vi "Main Data Log.vi"(8 "error in (no error)":errorcluster, 11 "main ref":T1) -> (0 "error out":errorcluster)   [LabVIEW 2025]
uses:
  controls/LAB-IQ UI Data.ctl
  Traction Loop/Traction Receipe Enum.ctl
panel:
  out "error out 2":errorcluster
  out "TDMS CLOSE":bool
  out "tdms file out":refnum<k34>
  out "File Create Temp":bool
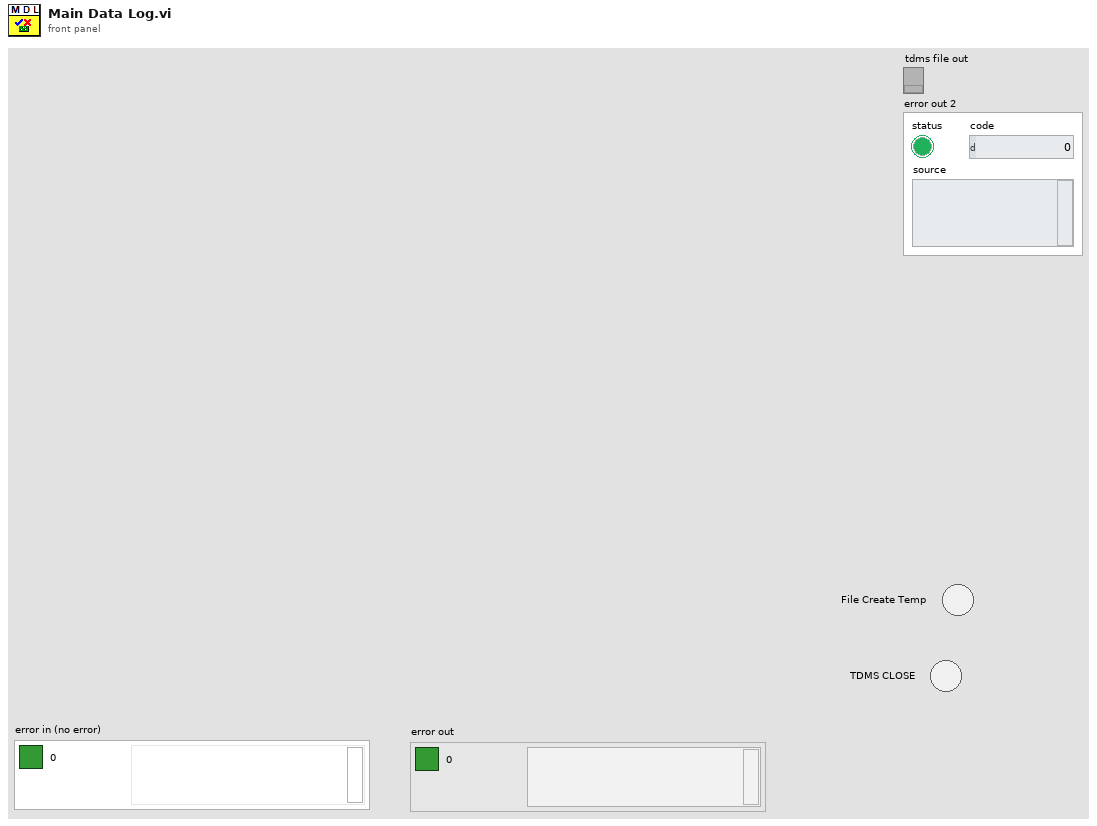
[diagram p1: front panel]
types:
  T1 = typedef "LAB-IQ UI Data.ctl" = cluster{"Main Home Screen":cluster{"GUI":refnum<vi>, "Platform Settings":refnum<vi>, "Configure":refnum<vi>, "Home":refnum<vi>, "EXIT":refnum<vi>, "service 2":refnum<vi>, "MainPage":refnum<vi>, "Analysis":refnum<vi>}, "Platform Settings":cluster{"mm/s  Surge":refnum<vi>, "Drive Error":refnum<vi>, "Disable Axis Jog Soft Limits":refnum<vi>, "mm/s  Sway":refnum<vi>, "Sway and Surge COM Status":refnum<vi>, "Heave COM Status":refnum<vi>, "Enable Platform":refnum<vi>, "Surge Forward Main":refnum<vi>, "Sway Right Main":refnum<vi>, "Sway Left Main":refnum<vi>, "Heave Down Main":refnum<vi>, "Heave Up main":refnum<vi>, "mm/s Heave":refnum<vi>, "mm/sec":refnum<vi>, "mm":refnum<vi>, "Surge Backward Main":refnum<vi>}, "Analysis Screen":cluster{"Analysis Home":refnum<vi>, "Surface Analysis":refnum<vi>, "Imaging":refnum<vi>, "Image Analysis":refnum<vi>, "Post Analysis":refnum<vi>}, "Config Screen":cluster{"Select Load Head":refnum<vi>, "Notes :":refnum<vi>, "FILE":refnum<vi>, "Sample ID :":refnum<vi>, "Operator ID :":refnum<vi>, "Operator Name :":refnum<vi>, "Auto":refnum<vi>}, "Motion Module":cluster{"zNL":refnum<vi>, "NL disp":refnum<vi>, "Rotary Tab":refnum<vi>, "Motion Direction:  3":refnum<vi>, "E.Velocity 2":refnum<vi>, "e.v/ssr 2":refnum<vi>, "Enter Fixed E.Velocity 2":refnum<vi>, "Enter Final SRR 2":refnum<vi>, "Enter initial SRR 2":refnum<vi>, "Enter Fixed SRR 2":refnum<vi>, "Enter the Final E.Velocity (m/s) 2":refnum<vi>, "Enter initial E.Velocity (m/s) 2":refnum<vi>, "Final Speed (RPM) 3":refnum<vi>, "Initial Speed (RPM) 2":refnum<vi>, "Enter the Final Velocity (m/s) 3":refnum<vi>, "Enter initial Velocity (m/s)  3":refnum<vi>, "Ramp Up 2":refnum<vi>, "TEST SELECTION":refnum<vi>, "SPEED SELECTION : ":refnum<vi>, "Angular Oscillation Set":refnum<vi>, "Traction":refnum<vi>, "Step Speed":refnum<vi>, "StepTable For Load-Speed":refnum<vi>, "StepTable For Speed":refnum<vi>, "Surge Forward MM":refnum<vi>, "Surge Backward MM":refnum<vi>, "M3 Image":refnum<vi>, "String 39":refnum<vi>, "Sway Left MM":refnum<vi>, "Sway Right MM":refnum<vi>, "Disable Axis Jog Soft Limits":refnum<vi>, "mm":refnum<vi>, "Heave Down MM":refnum<vi>, "Heave Up MM":refnum<vi>, "Wear Track Diameter (mm)":refnum<vi>, "Set WTD":refnum<vi>, "HomeScratch":refnum<vi>, "HomeRot":refnum<vi>, "PlaceModule":refnum<vi>, "Enter the Angle (Deg)":refnum<vi>, "Enter the Frequency (Hz)":refnum<vi>, "Motion Mode:":refnum<vi>, "LR Sway":refnum<vi>, "Rot Hor":refnum<vi>, "Scratch":refnum<vi>, "LR Cam":refnum<vi>, "MMBack":refnum<vi>, "MMNext":refnum<vi>, "Rot Ver":refnum<vi>, "Rotary Module Selection":refnum<vi>, "calculate rotary":refnum<vi>, "SPEED SELECTION : rotary":refnum<vi>, "Import 2":refnum<vi>, "Save 2":refnum<vi>, "File Path :  2":refnum<vi>, "String 45":refnum<vi>, "StepTable For Speed 3":refnum<vi>, "Enter the Speed(mm/sec)":refnum<vi>, "Enter the Speed(RPM)":refnum<vi>, "Enter Scratch Speed (mm/s):":refnum<vi>, "SwaySpeed Set":refnum<vi>, "Scartch Offset":refnum<vi>, "Motion type:":refnum<vi>, "HomeScratch 2":refnum<vi>, "Enter Scratch length (mm):":refnum<vi>, "Wear Track Diameter":refnum<vi>, "Rotary Speed Exced":refnum<vi>, "Scratch Mode":refnum<vi>, "No of Scratch":refnum<vi>}, "Environmental control":cluster{"Humidity  Status  3":refnum<vi>, "Low Temp  Status  2":refnum<vi>, "TK4 status 2":refnum<vi>, "Stage Temperature":refnum<vi>, "Sample Temperature":refnum<vi>, "Humidity (Amb)":refnum<vi>, "Clear List":refnum<vi>, "Add to list":refnum<vi>, "Wear":refnum<vi>, "Vibration":refnum<vi>, "Humidity (Chamber)":refnum<vi>, "Temperature (Chamber)":refnum<vi>, "ECR ":refnum<vi>, "Temperature (Amb)":refnum<vi>, "Microphone":refnum<vi>, "Acoustic Emission 3":refnum<vi>, "SNext":refnum<vi>, "APBack":refnum<vi>, "Enter the Temperature (°C):":refnum<vi>, "Enter the Stage \nTemperature (°C):":refnum<vi>, "Enter the Humidity (%Rh):":refnum<vi>, "Low Temp":refnum<vi>, "High Temp":refnum<vi>, "Humidity":refnum<vi>, "Sensors Picked":refnum<vi>}, "About Screen":cluster{"Password":refnum<vi>, "Home Service":refnum<vi>, "Advanced Setting":refnum<vi>, "About Tab":refnum<vi>, "ECR Port:":refnum<vi>, "Ramp Port:":refnum<vi>, "Installation/Replacement completed":refnum<vi>, "Loahead":refnum<vi>, "Heave and Surge COM Port:":refnum<vi>, "Sway COM Port:":refnum<vi>, "Temp Modbus:":refnum<vi>, "Humidity Port:":refnum<vi>, "Edit Gain Constants":refnum<vi>, "Save Gain Constants":refnum<vi>}, "Main Screen":cluster{"Main Screen Tab":refnum<vi>, "Angle and Frequency":refnum<vi>, "Stroke (mm)":refnum<vi>, "Angle (Deg)":refnum<vi>, "Main Speed Tab":refnum<vi>, "MTM MOTOR DISPLAY":refnum<vi>, "Disc Speed (m/sec)":refnum<vi>, "Ball Speed (m/sec)":refnum<vi>, "Disc Speed (RPM)":refnum<vi>, "Ball Speed (RPM)":refnum<vi>, "SPEED TAB":refnum<vi>, "Speed (m/sec)":refnum<vi>, "Set Speed (m/sec)":refnum<vi>, "Speed (RPM)":refnum<vi>, "Set Speed":refnum<vi>, "Time Tab":refnum<vi>, "Time ( HH:MM:SS ) 2":refnum<vi>, "Test Duration":refnum<vi>, "Test Duration 4":refnum<vi>, "TEST CYCLE":refnum<vi>, "TOTAL CYCLES":refnum<vi>, "Set Load (N)":refnum<vi>, "Temp Tabs":refnum<vi>, "Heater":refnum<vi>, "TK4 status":refnum<vi>, "ChamberTemp":refnum<vi>, "SetTmp":refnum<vi>, "Controller  Status":refnum<vi>, "ChamberTemp 2":refnum<vi>, "SetTmp 2":refnum<vi>, "Controller  Status 2":refnum<vi>, "ChamberTemp 3":refnum<vi>, "SetTmp 3":refnum<vi>, "Cooling":refnum<vi>, "Load Communication":refnum<vi>, "Ambient \nTemperature":refnum<vi>, "HumCOMStatus":refnum<vi>, "Ambient\n Humidity":refnum<vi>, "Freq (Hz)":refnum<vi>, "Load En":refnum<vi>, "NLt":refnum<vi>, "zNL 2":refnum<vi>, "Humidity On":refnum<vi>, "humidity disp":refnum<vi>, "Set Humidity":refnum<vi>, "NL disp 2":refnum<vi>, "Humidity On 2":refnum<vi>, "humidity disp 2":refnum<vi>, "Set Humidity 2":refnum<vi>, "NL disp 3":refnum<vi>, "AppLoadSeq scratch":refnum<vi>, "Stop Scratch":refnum<vi>, "ClrLog":refnum<vi>, "Trip Log":refnum<vi>, "STOP":refnum<vi>, "Start Test":refnum<vi>, "Test status":refnum<vi>, "AR Led":refnum<vi>, "Data":refnum<vi>, "Health":refnum<vi>, "Sway COM Status":refnum<vi>, "Heave COM Status":refnum<vi>, "Grp Tab":refnum<vi>, "Sub Graph":refnum<vi>, "SD (mm)":refnum<vi>, "Siliding distance Reset Graph":refnum<vi>, "SDGp":refnum<vi>, "Humidity Reset Graph":refnum<vi>, "HumrGp":refnum<vi>, "Acoustic Emission (mV)":refnum<vi>, "Aqucostic Reset Graph":refnum<vi>, "gACQUOS":refnum<vi>, "ECR RESET":refnum<vi>, "ECR":refnum<vi>, "Temperature Reset":refnum<vi>, "Acoustic Emission (mV) 2":refnum<vi>, "Aqucostic Reset Graph 2":refnum<vi>, "gACQUOS 2":refnum<vi>, "ECR RESET 2":refnum<vi>, "ECR 2":refnum<vi>, "Temperature Reset 2":refnum<vi>, "Temperature (deg c)":refnum<vi>, "Speed Reset Graph":refnum<vi>, "Speed Tab":refnum<vi>, "MTM DISC  SPEED":refnum<vi>, "MTM BALL SPEED":refnum<vi>, "speed mm/sec":refnum<vi>, "Hymidity":refnum<vi>, "Humidity Disable trip":refnum<vi>, "CoF Trip  2":refnum<vi>, "Depth Trip":refnum<vi>, "Weart Deapth":refnum<vi>, "Depth Reset Graph":refnum<vi>, "Weart":refnum<vi>, "Depthz":refnum<vi>, "Depth (µm)":refnum<vi>, "WearGp":refnum<vi>, "NL Trip 2":refnum<vi>, "Load pid":refnum<vi>, "Load Disable Trip":refnum<vi>, "Load Reset Graph":refnum<vi>, "NL Display 4":refnum<vi>, "Main Chart 3":refnum<vi>, "BACK":refnum<vi>, "Depth Trip 2":refnum<vi>, "COF TRIP ":refnum<vi>, "Friction Force (N)":refnum<vi>, "FF Reset Graph":refnum<vi>, "FF Disable Trip":refnum<vi>, "FF TRIP":refnum<vi>, "COF Disable Trip":refnum<vi>, "COF Reset Graph":refnum<vi>, "Start Test Temp":refnum<vi>, "zFF":refnum<vi>, "Friction Force (N) Graph":refnum<vi>, "Coefficient of Friction":refnum<vi>, "Scratch Start Test":refnum<vi>, "FF Tab":refnum<vi>, "Cyclic Friction Force (N)":refnum<vi>, "CZ FF":refnum<vi>, "Cyclic Friction Force (N) Graph":refnum<vi>, "Cyclic Coefficient of Friction":refnum<vi>, "Cyclic FF TRIP":refnum<vi>, "Cyclic FF Disable Trip":refnum<vi>, "cyclic COF Disable Trip":refnum<vi>, "cyclic COF TRIP":refnum<vi>, "cyclic COF Reset Graph":refnum<vi>, "Cyclic FF Reset Graph":refnum<vi>, "Test Trip":refnum<vi>, "Multi Scratch Pass":refnum<vi>, "Scratch Start Recording":refnum<vi>}, "Loading":cluster{"Indentation":refnum<vi>, "Reference Sample":refnum<vi>, "Load Cell Communication Slide":refnum<vi>, "com 3":refnum<vi>, "com":refnum<vi>, "DecaForce COM Status":refnum<vi>, "Update":refnum<vi>, "Clear 3":refnum<vi>, "seq":refnum<vi>, "Stribeck table":refnum<vi>, "Stribeck Table  For loading":refnum<vi>, "Loading Mode":refnum<vi>, "Enter the Final Load (N)":refnum<vi>, "Enter the CoF Trip":refnum<vi>, "Enter the Friction Force Trip":refnum<vi>, "Enter the Normal load Trip":refnum<vi>, "Enter the Load  (N)":refnum<vi>, "KiloForce":refnum<vi>, "DecaForce ":refnum<vi>, "MicroForce":refnum<vi>, "LHBack":refnum<vi>, "LHNext":refnum<vi>, "Enter the Loading Rate (N/min)":refnum<vi>, "Message":refnum<vi>, "Warning 2":refnum<vi>, "SSP 0.75":refnum<vi>, "SSP 0.5":refnum<vi>, "SSP 0.3":refnum<vi>, "Warning":refnum<vi>, "gui GIF":refnum<vi>, "Communication is established":refnum<vi>, "AppLoad 4":refnum<vi>, "Multipoint":refnum<vi>, "Load Selection":refnum<vi>}, "PID":cluster{"Ramp":refnum<vi>, "Vertical load (N)":refnum<vi>, "apply load":refnum<vi>, "apply load 2":refnum<vi>, "Enter ByPass Load":refnum<vi>, "Bypass Load":refnum<vi>, "gFF Rot":refnum<vi>}, "Config Parameters":cluster{"Tab Control 3":refnum<vi>, "Tab Control 19":refnum<vi>, "SAMPLES":refnum<vi>, "Re-initilaize":refnum<vi>, "Filter ON/OFF":refnum<vi>, "TracHomeSurgeOffsetCounts 10MM":refnum<vi>, "TracHomeSwayOffsetCounts 10MM":refnum<vi>, "Acoustic Emission:":refnum<vi>, "Apply Filter (FF)":refnum<vi>, "Filter% 2":refnum<vi>, "Apply Filter (Load)":refnum<vi>, "Filter% ":refnum<vi>, "Sway distance (mm)":refnum<vi>, "Surge distance (mm)":refnum<vi>, "DataSavingLoopDelay(ms)":refnum<vi>, "SAVE 2":refnum<vi>, "Enter Distance":refnum<vi>, "Sway Counts:":refnum<vi>, "Distance (mm): 3":refnum<vi>, "Surge Counts:":refnum<vi>, "Distance (mm): 2":refnum<vi>, "Distance (mm):":refnum<vi>, "Heave Counts:":refnum<vi>, "LRMHomeSurgeOffsetCounts":refnum<vi>, "LRMHomeSwayOffsetCounts":refnum<vi>, "TracHomeSurgeOffsetCounts 20MM":refnum<vi>, "TracHomeSwayOffsetCounts 20MM":refnum<vi>, "RotHomeSwayOffsetCounts":refnum<vi>, "RotHomeSurgeOffsetCounts":refnum<vi>, "Heave distance":refnum<vi>, "Zmm":refnum<vi>, "Heave Pulses/mm":refnum<vi>, "Surge Pulses/mm":refnum<vi>, "Sway Pulses/mm":refnum<vi>, "Heave Pitch":refnum<vi>, "Surge Pitch":refnum<vi>, "Sway Pitch":refnum<vi>, "Heave PPR":refnum<vi>, "Surge PPR":refnum<vi>, "Sway PPR":refnum<vi>, "Tab Control 5":refnum<vi>, "Tab Control 14":refnum<vi>, "Tab Control 26":refnum<vi>, "AE":refnum<vi>, "Heave Loop Delay":refnum<vi>, "Heave PID Speed":refnum<vi>, "Surge Jog Speed":refnum<vi>, "Heave Jog Speed":refnum<vi>, "Sway Loop Delay":refnum<vi>, "Sway PID Speed":refnum<vi>, "Sway Jog Speed":refnum<vi>, "DEPTH TRIP VALUE":refnum<vi>, "LOAD TRIP VALUE":refnum<vi>, "DEPTH TRIP   ENABLE":refnum<vi>, "LOAD TRIP  ENABLE":refnum<vi>, "CYCLIC FF TRIP VALUE":refnum<vi>, "FF TRIP VALUE":refnum<vi>, "CYCLIC CoF TRIP VALUE":refnum<vi>, "COF TRIP VALUE":refnum<vi>, "CYCLIC COF TRIP  ENABLE":refnum<vi>, "CYCLIC FF TRIP  ENABLE":refnum<vi>, "FF TRIP  ENABLE":refnum<vi>, "COF TRIP  ENABLE":refnum<vi>, "JOG TRIP LOAD VALUE (N)":refnum<vi>, "Rotary Vertical":refnum<vi>, "Traction":refnum<vi>, "Scratch":refnum<vi>, "LRM CAM":refnum<vi>, "Sway LRM":refnum<vi>, "Rotary Horizontal":refnum<vi>}, "Loading Com Port":cluster{"ClearAll":refnum<vi>, "Mz(Nm)":refnum<vi>, "My(Nm)":refnum<vi>, "Mx(Nm)":refnum<vi>, "Save Dwell":refnum<vi>, "Acq Delay (ms)":refnum<vi>, "Burst Delay (ms)":refnum<vi>, "model":refnum<vi>, "SN":refnum<vi>, "FFx(N)":refnum<vi>, "Sensor IP":refnum<vi>, "Port":refnum<vi>, "FFy(N)":refnum<vi>, "Load(N)":refnum<vi>, "delete Handle":refnum<vi>, "Create Handle":refnum<vi>, "ft_data":refnum<vi>, "ft_range":refnum<vi>, "ft_data 2":refnum<vi>, "stop 6":refnum<vi>, "running_flag":refnum<vi>, "ft_udp_handle":refnum<vi>, "get-data-return":refnum<vi>, "get-range-return":refnum<vi>, "zero-return":refnum<vi>, "filter-return":refnum<vi>, "initial-return":refnum<vi>, "deleteHandle-result":refnum<vi>, "Load Cell Temp":refnum<vi>, "Load Cell":refnum<vi>, "ZeroAll":refnum<vi>, "FORCE (N)":refnum<vi>, "TORQUE (N-m)":refnum<vi>}, "Heave AND Surge":cluster{"SURGE POSE":refnum<vi>, "error out Read":refnum<vi>, "HEAVE POSE":refnum<vi>, "State":refnum<vi>, "Homed":refnum<vi>, "Sequence ID":refnum<vi>, "error out Write":refnum<vi>, "faultCode":refnum<vi>, "Ack ID":refnum<vi>, "SPEED":refnum<vi>, "Distance":refnum<vi>, "Mode Command":refnum<vi>, "Heave and Surge Read":refnum<vi>, "Read Heave Temp":refnum<vi>, "Spare 15":refnum<vi>, "Spare 14":refnum<vi>, "Spare 13":refnum<vi>, "Spare 12":refnum<vi>, "Spare 11":refnum<vi>, "Spare 10":refnum<vi>, "Spare 9":refnum<vi>, "Spare 8":refnum<vi>, "Spare 7":refnum<vi>, "Spare 4":refnum<vi>, "Spare 3":refnum<vi>, "Spare 2":refnum<vi>, "Humidity":refnum<vi>, "Temp":refnum<vi>, "Node Id":refnum<vi>, "Spare 1":refnum<vi>, "SPARE 4":refnum<vi>, "SPARE 3":refnum<vi>, "SPARE 2":refnum<vi>, "SPARE 1":refnum<vi>, "fwMajor":refnum<vi>, "fwMinor":refnum<vi>, "Manual Write":refnum<vi>, "Heave and Surge Write":refnum<vi>, "SPARE 5":refnum<vi>, "Reserved ":refnum<vi>, "SPARE 8":refnum<vi>, "SPARE 6":refnum<vi>, "SPARE 7":refnum<vi>, "SPARE 17":refnum<vi>, "SPARE 16":refnum<vi>, "SPARE 15":refnum<vi>, "SPARE 14":refnum<vi>, "SPARE 13":refnum<vi>, "SPARE 12":refnum<vi>, "SPARE 11":refnum<vi>, "SPARE 10":refnum<vi>, "SPARE 9":refnum<vi>, "System UPTIME":refnum<vi>, "Missed Packets":refnum<vi>, "faultCode Surge Right":refnum<vi>, "faultCode Surge Left":refnum<vi>, "faultCode Heave":refnum<vi>, "UPLINK HEAVE":refnum<vi>, "DOWNLINK HEAVE":refnum<vi>}, "New PID LOGIC":cluster{"Fine Tune Zone":refnum<vi>, "PID SDelay":refnum<vi>, "Max_pos_limit":refnum<vi>, "Min_pos_limit":refnum<vi>, "i_limit":refnum<vi>, "pct_scale":refnum<vi>, "Deadband":refnum<vi>, "Kd":refnum<vi>, "Ki":refnum<vi>, "Kp":refnum<vi>, "Current Position":refnum<vi>, "Set Load":refnum<vi>, "Current Load":refnum<vi>, "Pulse delta":refnum<vi>, "Init Step":refnum<vi>, "Max Step Linit":refnum<vi>, "min_deadband_floor":refnum<vi>, "dynamic_spindle_noise_scalar":refnum<vi>, "min_finetune_floor":refnum<vi>, "filter_alpha":refnum<vi>, "PID":refnum<vi>}, "SWAY ":cluster{"fwMajor":refnum<vi>, "Homed":refnum<vi>, "Rotary POSE":refnum<vi>, "State":refnum<vi>, "SWAY POSE":refnum<vi>, "Ack ID":refnum<vi>, "faultCode":refnum<vi>, "Node Id":refnum<vi>, "fwMinor":refnum<vi>, "Spare 6":refnum<vi>, "Spare 5":refnum<vi>, "Spare 4":refnum<vi>, "Spare 3":refnum<vi>, "Spare 2":refnum<vi>, "Spare 1":refnum<vi>, "Spare 7":refnum<vi>, "SPARE  5":refnum<vi>, "error out Write  SWAY ":refnum<vi>, "error out Read SWAY ":refnum<vi>, "Manual Write SWAY ":refnum<vi>, "SWAY WRITE":refnum<vi>, "SPARE  4":refnum<vi>, "SPARE  3":refnum<vi>, "SPARE 2":refnum<vi>, "SPARE 1":refnum<vi>, "Spare 15":refnum<vi>, "Spare 14":refnum<vi>, "Spare 13":refnum<vi>, "Spare 12":refnum<vi>, "Spare 11":refnum<vi>, "Spare 9":refnum<vi>, "Spare 8":refnum<vi>, "SPEED":refnum<vi>, "Distance":refnum<vi>, "Mode Command":refnum<vi>, "Sequence ID":refnum<vi>, "SWAY READ":refnum<vi>, "Spare 10":refnum<vi>, "Read SWAY Temp":refnum<vi>, "faultCode Sway ":refnum<vi>, "Missed Packets":refnum<vi>, "System UPTIME sway":refnum<vi>, "SPARE 6":refnum<vi>, "SPARE 7":refnum<vi>, "SPARE 9":refnum<vi>, "SPARE 11":refnum<vi>, "SPARE 10":refnum<vi>, "SPARE 8":refnum<vi>, "SPARE 13":refnum<vi>, "SPARE 12":refnum<vi>, "SPARE 17":refnum<vi>, "SPARE 16":refnum<vi>, "SPARE 15":refnum<vi>, "SPARE 14":refnum<vi>, "Reserved":refnum<vi>, "faultCode Rotary":refnum<vi>, "UPLINK SWAY":refnum<vi>, "DOWNLINK SWAY":refnum<vi>}, "Analysis Screen":cluster{"Analysis Home":refnum<vi>, "Refresh 2":refnum<vi>, "MEAN 4":refnum<vi>, "SD 4":refnum<vi>, "VARIANCE 4":refnum<vi>, "MEAN  3":refnum<vi>, "SD  3":refnum<vi>, "VARIANCE  3":refnum<vi>, "MEAN 2":refnum<vi>, "SD  2":refnum<vi>, "VARIANCE 2":refnum<vi>, "MEAN":refnum<vi>, "SD":refnum<vi>, "VARIANCE":refnum<vi>, "File 4 Discription":refnum<vi>, "OPEN 4":refnum<vi>, "File Name 4":refnum<vi>, "OPEN 3":refnum<vi>, "File 3 Discription":refnum<vi>, "File Name 3":refnum<vi>, "Y-AXIS":refnum<vi>, "X-AXIS":refnum<vi>, "XY Graph":refnum<vi>, "File Name 2":refnum<vi>, "File Name 1":refnum<vi>, "OPEN 2":refnum<vi>, "OPEN 1":refnum<vi>, "File 1 Discription ":refnum<vi>, "File 2 Discription":refnum<vi>, "Export":refnum<vi>, "File Format":refnum<vi>}, "Traction":cluster{"faultCode Traction 2":refnum<vi>, "faultCode Traction 1":refnum<vi>, "Missed Packets":refnum<vi>, "System UPTIME Traction":refnum<vi>, "SPARE 17":refnum<vi>, "SPARE 16":refnum<vi>, "SPARE 15":refnum<vi>, "SPARE 14":refnum<vi>, "SPARE 13":refnum<vi>, "SPARE 12":refnum<vi>, "SPARE 11":refnum<vi>, "SPARE 10":refnum<vi>, "SPARE 9":refnum<vi>, "SPARE 8":refnum<vi>, "SPARE 7":refnum<vi>, "SPARE 6":refnum<vi>, "Reserved":refnum<vi>, "SPARE  5":refnum<vi>, "Manual Write TRACTION":refnum<vi>, "TRACTION WRITE":refnum<vi>, "SPARE  4":refnum<vi>, "SPARE  3":refnum<vi>, "SPARE 2":refnum<vi>, "SPARE 1":refnum<vi>, "Spare 7":refnum<vi>, "Spare 6":refnum<vi>, "Spare 5":refnum<vi>, "Spare 4":refnum<vi>, "Spare 2":refnum<vi>, "Spare 1":refnum<vi>, "Node Id":refnum<vi>, "Read TRACTION Temp":refnum<vi>, "fwMinor":refnum<vi>, "fwMajor":refnum<vi>, "faultCode":refnum<vi>, "TRACTION POSE":refnum<vi>, "TRACTION POSE 2":refnum<vi>, "Homed":refnum<vi>, "State":refnum<vi>, "Ack ID":refnum<vi>, "SPEED":refnum<vi>, "Distance":refnum<vi>, "Mode Command":refnum<vi>, "Sequence ID":refnum<vi>, "error out Read TRACTION":refnum<vi>, "error out Write  TRACTION":refnum<vi>, "TRACTION READ":refnum<vi>, "Spare 3":refnum<vi>, "Downlink traction":refnum<vi>, "Uplink Traction":refnum<vi>}, "Traction reciepe":cluster{"SRR Sweep Range (%) Stribeck":refnum<vi>, "Traction Receipe":refnum<vi>, "Total Execution Time":refnum<vi>, "Total Steps":refnum<vi>, "Duration / Step (s)  Stribeck":refnum<vi>, "STRIBECK Fixed SRR List (%)":refnum<vi>, "Duration / Step (s) Traction":refnum<vi>, "SRR Sweep Range (%) traction":refnum<vi>, "Rolling Speed (mm/s)":refnum<vi>, "Temperature Stages (°C)":refnum<vi>, "Ball Load (N)":refnum<vi>, "Lubricant Name":refnum<vi>, "Profile File Name":refnum<vi>, "SET entrainment Velocity":refnum<vi>, "Test Array Size":refnum<vi>, "SRR INDEX [ STRIBECK]":refnum<vi>, "Stribeck Size":refnum<vi>, "SET SRR":refnum<vi>, "ELAPSED TIMER ":refnum<vi>, "BALL SET RPM":refnum<vi>, "DISC SET RPM":refnum<vi>, "SET LOAD":refnum<vi>, "TEMPERATURE READ":refnum<vi>, "SET TEMPERATURE":refnum<vi>, "Traction Size":refnum<vi>, "DISC SPEED (rpm)":refnum<vi>, "BALL SPEED (rpm)":refnum<vi>, "BALL WEAR TRACK":refnum<vi>, "DISC WEARTRACK":refnum<vi>, "SRR INDEX [ TRACTION]":refnum<vi>, "Start Index Type":refnum<vi>, "Enum - Menu":refnum<vi>, "Ball (mm/sec)":refnum<vi>, "Disc (mm/sec)":refnum<vi>}, "Traction Control":cluster{"HomeTraction":refnum<vi>, "Demo Mode Display":refnum<vi>, "Traction Message":refnum<vi>, "Traction Step Update Details":refnum<vi>, "Main Tab sequence for selection":refnum<vi>, "Ramp Tab":refnum<vi>, "e.v/ssr":refnum<vi>, "Enter Fixed E.Velocity":refnum<vi>, "Enter Final SRR":refnum<vi>, "Enter initial SRR":refnum<vi>, "Enter Fixed SRR":refnum<vi>, "Enter the Final E.Velocity (m/s)":refnum<vi>, "Enter initial E.Velocity (m/s)":refnum<vi>, "Ball WTD":refnum<vi>, "E.Velocity":refnum<vi>, "Enter the Final Velocity (m/s)":refnum<vi>, "Enter initial Velocity (m/s)":refnum<vi>, "Ramp Up   Disc":refnum<vi>, "Initial DiscSpeed (RPM)":refnum<vi>, "Final Speed (RPM) Ball":refnum<vi>, "Final Speed (RPM)":refnum<vi>, "Initial Speed (RPM) Ball":refnum<vi>, "Enter the Final Velocity (m/s) Ball":refnum<vi>, "Enter initial Velocity (m/s) Ball":refnum<vi>, "Ramp Up":refnum<vi>, "ExceedBallSpeed step":refnum<vi>, "ExceedDiscSpeed":refnum<vi>, "BallSpeed Exceed Indication":refnum<vi>, "Apply":refnum<vi>, "SPEED SELECTION : MTM":refnum<vi>, "SPEED SELECTION : MTM 2":refnum<vi>, "TEST SELECTION (MTM)":refnum<vi>, "MTM Test Selection":refnum<vi>, "File Path Tab":refnum<vi>, "File Path String":refnum<vi>, "Save":refnum<vi>, "Save  2":refnum<vi>, "Import ":refnum<vi>, "File Path :":refnum<vi>, "Step Sequence Indication Tab":refnum<vi>, "Step Sequence Indication":refnum<vi>, "Calculate Step":refnum<vi>, "StepTable":refnum<vi>, "ExceedDiscSpeed  Cinstant Speed":refnum<vi>, "ExceedBallSpeed Constant":refnum<vi>, "TEST SELECTION (MTM) 2":refnum<vi>, "SPEED SELECTION : MTM 3":refnum<vi>, "MTM Test Selection 2":refnum<vi>, "Enter the Speed (m/sec): ":refnum<vi>, "Enter the Speed (m/sec):  2":refnum<vi>, "Enter the Speed (RPM):":refnum<vi>, "Lower Spped ":refnum<vi>, "Upper":refnum<vi>, "Enter the Speed (RPM):Ball":refnum<vi>, "Disc Motion Direction: ":refnum<vi>, "Ball Motion Direction :":refnum<vi>, "Motion Mode: ":refnum<vi>, "Wear Track Diameter (mm) ":refnum<vi>, "Disc Speed Indicator":refnum<vi>, "ExceedBallSpeed":refnum<vi>}, "Acquostic":cluster{"Last Config Rejected ":refnum<vi>, "rx command count":refnum<vi>, "Current Filter Id":refnum<vi>, "Isolated Gain":refnum<vi>, "DAQ Status":refnum<vi>, "error out":refnum<vi>, "error in (no error)":refnum<vi>, "Uplink Packet":refnum<vi>, "data out":refnum<vi>, "Downlink Packet":refnum<vi>, "Gains":refnum<vi>, "Manual Write Acquostic":refnum<vi>, "Acoustic Graphs":refnum<vi>}}
  T2 = enum32{"  Acquire  ", "Compare Files Rot", "About", "Service"}
  T3 = enum32{"Setup", "Load Head", "Motion Module", "Environment", "Begin"}
  T4 = enum16{"open", "open or create", "create or replace", "create", "open (read-only)"}
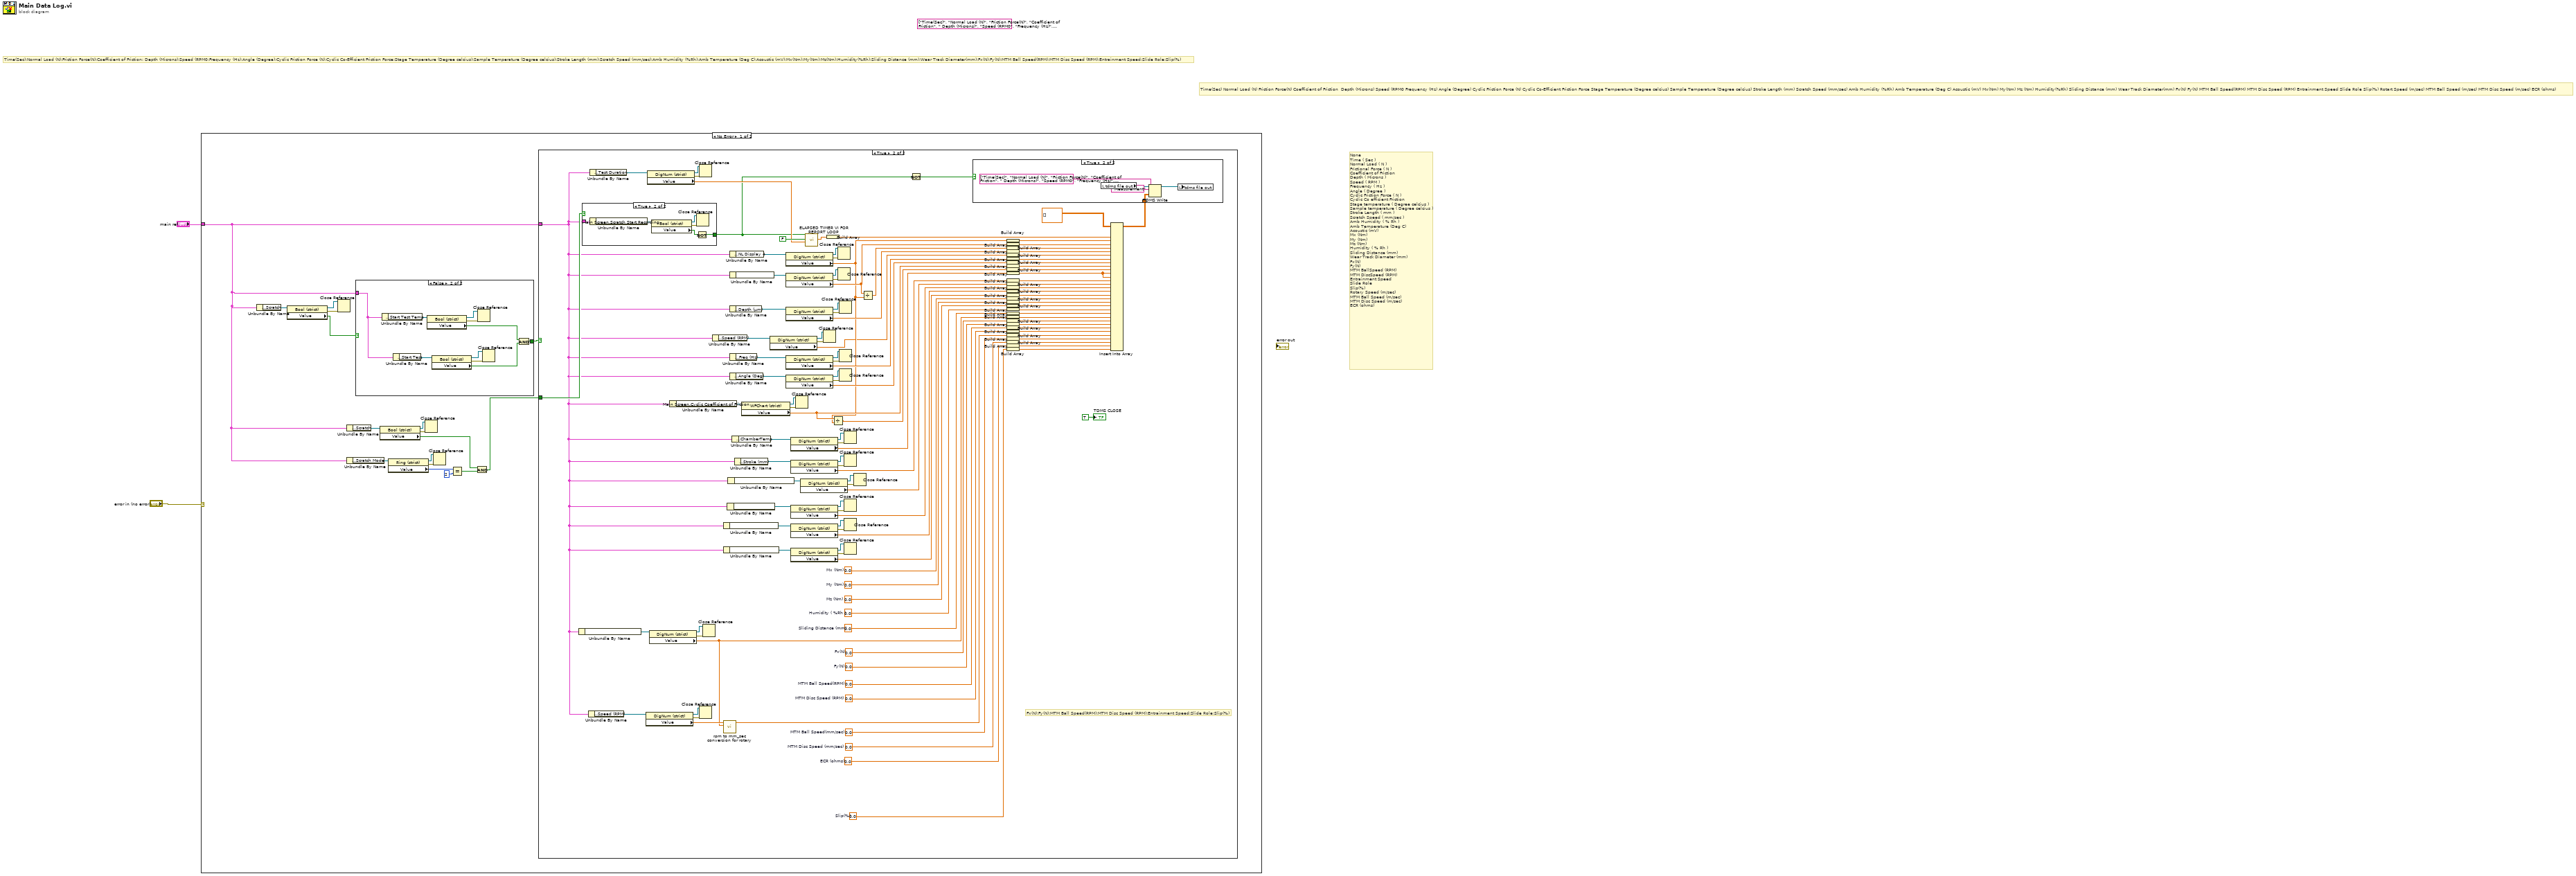
[diagram p0: block diagram]
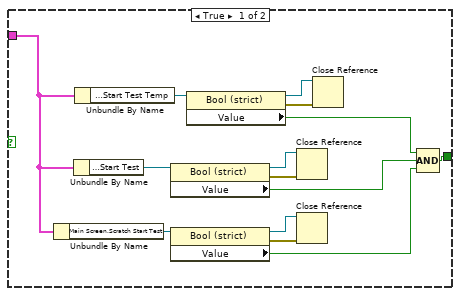
[diagram p2: hidden frame]
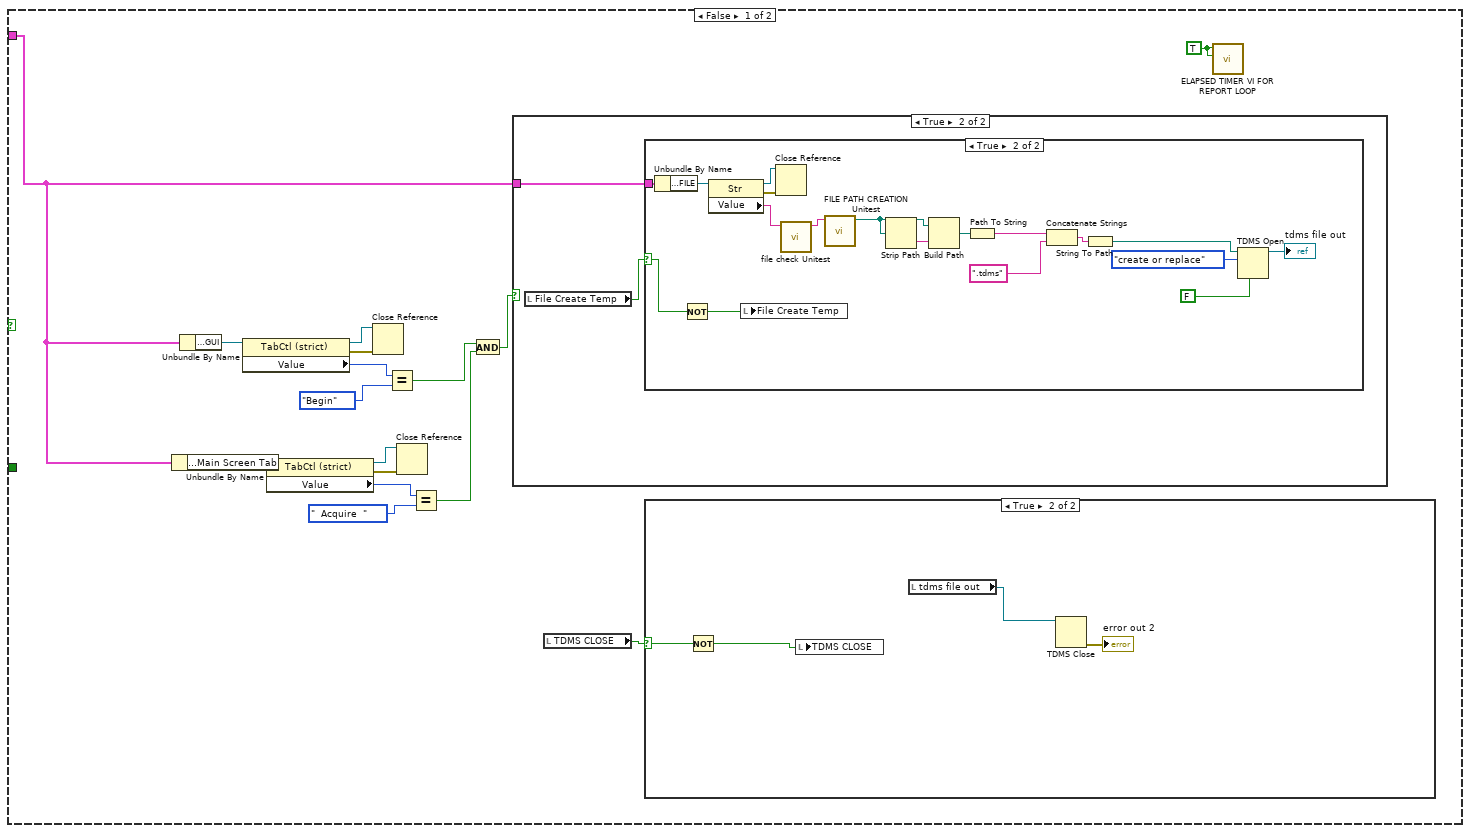
[diagram p3: hidden frame]
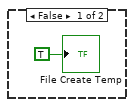
[diagram p5: hidden frame]
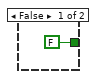
[diagram p7: hidden frame]
diagram:
  (unwired) string[] ["Time(Sec)", "Normal Load (N)", "Friction Force(N)", "Coefficient of Friction", " Depth (Microns)", "Speed (RPM0", "Frequency (Hz)", "Angle (Degree)", "Cyclic Friction Force (N)", "Cyclic Co-Efficient Friction Force", "Stage Temperature (Degree celcius)", "Sample Temperature (Degree celcius)", "Stroke Length (mm)", "Scratch Speed (mm/sec)", "Amb Humidity (%Rh)", "Amb Temperature (Deg C)", "Acoustic (mV)", "Mx(Nm)", "My(Nm)", "Mz (Nm)", "Humidity(%Rh)", "Sliding Distance (mm)", "Wear Track Diameter(mm)", "Fx(N)", "Fy(N)", "MTM Ball Speed(RPM)", "MTM Disc Speed (RPM)", "Entrainment Speed", "Slide Role", "Slip(%)", "Rotart Speed (m/sec)", "MTM Ball Speed (m/sec)", "MTM Disc Speed (m/sec)", "ECR (ohms)"] ("array")
  # "Time(Sec)\tNormal Load (N)\tFriction Force(N)\tCoefficient of Friction\t Depth (Microns)\tSpeed (RPM0\tFrequency (Hz)\tAngle (Degree)\tCyclic Friction Force (N)\tCyclic Co-Efficient Friction Force\tStage Temperature (Degree celcius)\tSample Temperature (Degree celcius)\tStroke Length (mm)\tScratch Speed (mm/sec)\tAmb Humidity (%Rh)\tAmb Temperature (Deg C)\tAcoustic (mV)\tMx(Nm)\tMy(Nm)\tMz (Nm)\tHumidity(%Rh)\tSliding Distance (mm)\tWear Track Diameter(mm)\tFx(N)\tFy(N)\tMTM Ball Speed(RPM)\tMTM Disc Speed (RPM)\tEntrainment Speed\tSlide Role\tSlip(%)\tRotart Speed (m/sec)\tMTM Ball Speed (m/sec)\tMTM Disc Speed (m/sec)\tECR (ohms)"
  # "None\t\nTime ( Sec )\t\nNormal Load ( N )\t\nFrictional Force ( N )\t\nCoefficient of Friction\t\nDepth ( Microns )\t\nSpeed ( RPM )\t\nFrequency ( Hz )\t\nAngle ( Degree )\t\nCyclic Friction Force ( N )\t\nCyclic Co efficient Friction \t\nStage temperature ( Degree celcius )\t\nSample temperature ( Degree celcius )\t\nStroke Length ( mm )\t\nScratch Speed ( mm/sec )\t\nAmb Humidity ( % Rh ) \t\nAmb Temperature (Deg C)\t\nAcoustic (mV)\t\nMx (Nm)\t\nMy (Nm)\t\nMz (Nm)\t\nHumidity ( % Rh )\t\nSliding Distance (mm)\t\nWear Track Diameter (mm)\t\nFx(N)\t\nFy(N)\t\nMTM BallSpeed (RPM)\t\nMTM DiscSpeed (RPM)\t\nEntrainment Speed\t\nSlide Role\t\nSlip(%)\t\nRotary Speed (m/sec)\t\nMTM Ball Speed (m/sec)\t\nMTM Disc Speed (m/sec)\t\nECR (ohms)"
  # "Time(Sec):Normal Load (N):Friction Force(N):Coefficient of Friction: Depth (Microns):Speed (RPM0:Frequency (Hz):Angle (Degree):Cyclic Friction Force (N):Cyclic Co-Efficient Friction Force:Stage Temperature (Degree celcius):Sample Temperature (Degree celcius):Stroke Length (mm):Scratch Speed (mm/sec):Amb Humidity (%Rh):Amb Temperature (Deg C):Acoustic (mV):Mx(Nm):My(Nm);Mz(Nm):Humidity(%Rh):Sliding Distance (mm):Wear Track Diameter(mm):Fx(N):Fy(N):MTM Ball Speed(RPM):MTM Disc Speed (RPM):Entrainment Speed:Slide Role:Slip(%)"
  n1 = case shown="No Error" "error in (no error)" {
    tunnel: "main ref" -> [w4 _]
    frame No Error {
      n2 = Unbundle By Name(w4) -> ("Motion Module.Scratch"=w18:refnum<vi>)
      n3 = property class="Bool (strict)"(reference=w18) -> (reference out=w19:refnum<vi>, error out=w17:errorcluster, "Value"=w16:bool)  [unwired: 1 in]
      n4 = Close Reference(reference=w19, error in (no error)=w17) -> ()  [unwired: 1 out]
      n5 = Unbundle By Name(w4) -> ("Motion Module.Scratch"=w13:refnum<vi>)
      n6 = Unbundle By Name(w4) -> ("Motion Module.Scratch Mode"=w10:refnum<vi>)
      n7 = case shown="False" w16 {
        tunnel: w4 -> [w21 w37]
        tunnel: [w25 w34] -> w15
        frame True {
          n8 = Unbundle By Name(w21) -> ("Main Screen.Scratch Start Test"=w23:refnum<vi>)
          n9 = Unbundle By Name(w21) -> ("Main Screen.Start Test"=w29:refnum<vi>)
          n10 = Unbundle By Name(w21) -> ("Main Screen.Start Test Temp"=w32:refnum<vi>)
          n11 = property class="Bool (strict)"(reference=w29) -> (reference out=w28:refnum<vi>, error out=w30:errorcluster, "Value"=w26:bool)  [unwired: 1 in]
          n12 = property class="Bool (strict)"(reference=w23) -> (reference out=w24:refnum<vi>, error out=w22:errorcluster, "Value"=w20:bool)  [unwired: 1 in]
          n13 = property class="Bool (strict)"(reference=w32) -> (reference out=w33:refnum<vi>, error out=w31:errorcluster, "Value"=w27:bool)  [unwired: 1 in]
          n14 = Close Reference(reference=w28, error in (no error)=w30) -> ()  [unwired: 1 out]
          n15 = Close Reference(reference=w24, error in (no error)=w22) -> ()  [unwired: 1 out]
          n16 = Close Reference(reference=w33, error in (no error)=w31) -> ()  [unwired: 1 out]
          n17 = Compound Arithmetic op=AND(w27, w26, w20) -> (w25:bool)
        }
        frame False {
          n18 = Unbundle By Name(w37) -> ("Main Screen.Start Test Temp"=w42:refnum<vi>)
          n19 = Unbundle By Name(w37) -> ("Main Screen.Start Test"=w39:refnum<vi>)
          n20 = property class="Bool (strict)"(reference=w42) -> (reference out=w43:refnum<vi>, error out=w41:errorcluster, "Value"=w36:bool)  [unwired: 1 in]
          n21 = property class="Bool (strict)"(reference=w39) -> (reference out=w38:refnum<vi>, error out=w40:errorcluster, "Value"=w35:bool)  [unwired: 1 in]
          n22 = Close Reference(reference=w43, error in (no error)=w41) -> ()  [unwired: 1 out]
          n23 = Close Reference(reference=w38, error in (no error)=w40) -> ()  [unwired: 1 out]
          n24 = And(x=w36, y=w35) -> (x .and. y?=w34:bool)
        }
      }
      n25 = property class="Bool (strict)"(reference=w13) -> (reference out=w12:refnum<vi>, error out=w14:errorcluster, "Value"=w5:bool)  [unwired: 1 in]
      n26 = property class="Ring (strict)"(reference=w10) -> (reference out=w11:refnum<vi>, error out=w9:errorcluster, "Value"=w8:u16)  [unwired: 1 in]
      n27 = Close Reference(reference=w12, error in (no error)=w14) -> ()  [unwired: 1 out]
      n28 = Close Reference(reference=w11, error in (no error)=w9) -> ()  [unwired: 1 out]
      n29 = Equal?(x=w8, y=u16 2) -> (x = y?=w6:bool)
      n30 = Compound Arithmetic op=AND(w5, w6) -> (w3:bool)
      n31 = case shown="True" w15 {
        tunnel: w4 -> [w49 w101]
        tunnel: w3 -> [_ w117]
        frame False {
          w59 = TRUE ("PAUSE")
          n32 = Unbundle By Name(w49) -> ("Main Screen.Main Screen Tab"=w51:refnum<vi>)
          n33 = Unbundle By Name(w49) -> ("Main Home Screen.GUI"=w57:refnum<vi>)
          n34 = property class="TabCtl (strict)"(reference=w57) -> (reference out=w56:refnum<vi>, error out=w58:errorcluster, "Value"=w55:T3)  [unwired: 1 in]
          n35 = property class="TabCtl (strict)"(reference=w51) -> (reference out=w52:refnum<vi>, error out=w50:errorcluster, "Value"=w53:T2)  [unwired: 1 in]
          n36 = Close Reference(reference=w56, error in (no error)=w58) -> ()  [unwired: 1 out]
          n37 = Equal?(x=w55, y=T3."Begin" ("Value")) -> (x = y?=w47:bool)
          n38 = Close Reference(reference=w52, error in (no error)=w50) -> ()  [unwired: 1 out]
          n39 = Equal?(x=w53, y=T2."  Acquire  " ("Value")) -> (x = y?=w46:bool)
          n40 = And(x=w47, y=w46) -> (x .and. y?=w45:bool)
          n41 = case shown="True" w45 {
            tunnel: w49 -> [_ w66]
            frame False {
              "File Create Temp" <- TRUE ("File Create Temp")
            }
            frame True {
              n42 = local read "File Create Temp"() -> (w65:bool)
              n43 = case shown="True" w65 {
                selector: w65 -> [_ w74]
                tunnel: w66 -> [_ w75]
                frame False {
                }
                frame True {
                  n44 = Unbundle By Name(w75) -> ("Config Screen.FILE"=w76:refnum<vi>)
                  n45 = Not(x=w74) -> (.not. x?=w73:bool)
                  n46 = property class="Str"(reference=w76) -> (reference out=w78:refnum<vi>, error out=w77:errorcluster, "Value"=w68:string)  [unwired: 1 in]
                  n47 = local write "File Create Temp"(w73) -> ()
                  n48 = Close Reference(reference=w78, error in (no error)=w77) -> ()  [unwired: 1 out]
                  n49 = call "file check Unitest.vi"("file name in"=w68) -> ("file name out"=w67:string)  [unwired: 9 in, 1 out]
                  n50 = call "FILE PATH CREATION Unitest.vi"("FILE NAME :"=w67) -> ("FILE OUT"=w79:path)  [unwired: 9 in, 1 out]
                  n51 = Strip Path(path=w79) -> (name=w82:string)  [unwired: 1 out]
                  n52 = Build Path(base path=w79, name or relative path=w82) -> (appended path=w83:path)
                  n53 = Path To String(path=w83) -> (string=w80:string)
                  n54 = Concatenate Strings(w80, ".tdms" ("string")) -> (w81:string)
                  n55 = String To Path(string=w81) -> (path=w70:path)
                  n56 = TDMS Open(6:FALSE ("disable buffering (T)"), 10:T4."create or replace" ("operation"), 11:w70) -> (3:→"tdms file out":refnum<k34>)  [unwired: 4 in, 1 out]
                }
              }
            }
          }
          n57 = local read "TDMS CLOSE"() -> (w44:bool)
          n58 = case shown="True" w44 {
            selector: w44 -> [_ w63]
            frame False {
            }
            frame True {
              n59 = Not(x=w63) -> (.not. x?=w62:bool)
              n60 = local write "TDMS CLOSE"(w62) -> ()
              n61 = local read "tdms file out"() -> (w61:refnum<k34>)
              n62 = TDMS Close(11:w61) -> (0:→"error out 2":errorcluster)  [unwired: 1 in, 1 out]
            }
          }
          n63 = call "ELAPSED TIMER VI FOR REPORT LOOP.vi"("RESET"=w59, "PAUSE"=w59) -> ()  [unwired: 7 in, 3 out]
        }
        frame True {
          w85 = 0.0  # Humidity ( %Rh )
          w105 = 0.0  # Fy(N)
          w106 = 0.0  # Fx(N)
          w150 = 0.0  # Slip(%)
          w151 = 0.0  # ECR (ohms)
          w152 = 0.0  # MTM Disc Speed (mm/sec)
          w153 = 0.0  # MTM Ball Speed(mm/sec)
          w154 = 0.0  # MTM Disc Speed (RPM)
          w155 = 0.0  # MTM Ball Speed(RPM)
          w156 = 0.0  # Mz (Nm)
          w157 = 0.0  # My (Nm)
          w158 = 0.0  # Mx (Nm)
          w86 = 0.0  # Sliding Distance (mm)
          # "Fx(N):Fy(N):MTM Ball Speed(RPM):MTM Disc Speed (RPM):Entrainment Speed:Slide Role:Slip(%)"
          n64 = Unbundle By Name(w101) -> ("Motion Module.Wear Track Diameter (mm)"=w166:refnum<vi>)
          n65 = case shown="True" w117 {
            tunnel: w101 -> [_ w208]
            tunnel: [FALSE ("Value") w206] -> w116
            frame False {
            }
            frame True {
              n66 = Unbundle By Name(w208) -> ("Main Screen.Scratch Start Recording"=w210:refnum<vi>)
              n67 = property class="Bool (strict)"(reference=w210) -> (reference out=w209:refnum<vi>, error out=w211:errorcluster, "Value"=w207:bool)  [unwired: 1 in]
              n68 = Not(x=w207) -> (.not. x?=w206:bool)
              n69 = Close Reference(reference=w209, error in (no error)=w211) -> ()  [unwired: 1 out]
            }
          }
          n70 = Unbundle By Name(w101) -> ("Main Screen.Speed (RPM)"=w102:refnum<vi>)
          n71 = Unbundle By Name(w101) -> ("Main Screen.Test Duration"=w147:refnum<vi>)
          n72 = property class="DigNum (strict)"(reference=w102) -> (reference out=w104:refnum<vi>, error out=w103:errorcluster, "Value"=w100:dbl)  [unwired: 1 in]
          n73 = property class="DigNum (strict)"(reference=w147) -> (reference out=w148:refnum<vi>, error out=w149:errorcluster, "Value"=w146:dbl)  [unwired: 1 in]
          n74 = property class="DigNum (strict)"(reference=w166) -> (reference out=w165:refnum<vi>, error out=w167:errorcluster, "Value"=w99:dbl)  [unwired: 1 in]
          n75 = Unbundle By Name(w101) -> ("Main Screen.Cyclic Coefficient of Friction"=w145:refnum<vi>)
          n76 = Close Reference(reference=w148, error in (no error)=w149) -> ()  [unwired: 1 out]
          n77 = Close Reference(reference=w104, error in (no error)=w103) -> ()  [unwired: 1 out]
          n78 = Close Reference(reference=w165, error in (no error)=w167) -> ()  [unwired: 1 out]
          n79 = Unbundle By Name(w101) -> ("Main Screen.Speed (RPM)"=w108:refnum<vi>)
          n80 = Unbundle By Name(w101) -> ("Main Screen.Acoustic Emission (mV)"=w163:refnum<vi>)
          n81 = Unbundle By Name(w101) -> ("Main Screen.Ambient \nTemperature"=w169:refnum<vi>)
          n82 = call "rpm to mm_sec conversion for rotary.vi"("Wear Track Diameter"=w99, "Initial Speed (RPM)"=w100) -> ("Enter initial Velocity (m/s)  4"=w98:dbl)  [unwired: 7 in, 2 out]
          n83 = Unbundle By Name(w101) -> ("Main Screen.Ambient\n Humidity"=w172:refnum<vi>)
          n84 = Unbundle By Name(w101) -> ("Motion Module.Enter Scratch Speed (mm/s):"=w113:refnum<vi>)
          n85 = Unbundle By Name(w101) -> ("Main Screen.NL Display 4"=w201:refnum<vi>)
          n86 = Unbundle By Name(w101) -> ("Main Screen.Friction Force (N)"=w196:refnum<vi>)
          n87 = Unbundle By Name(w101) -> ("Main Screen.Depth (µm)"=w193:refnum<vi>)
          n88 = Unbundle By Name(w101) -> ("Main Screen.Freq (Hz)"=w187:refnum<vi>)
          n89 = Unbundle By Name(w101) -> ("Main Screen.Angle (Deg)"=w186:refnum<vi>)
          n90 = Unbundle By Name(w101) -> ("Main Screen.ChamberTemp"=w182:refnum<vi>)
          n91 = Unbundle By Name(w101) -> ("Main Screen.Stroke (mm)"=w176:refnum<vi>)
          n92 = property class="WFChart (strict)"(reference=w145) -> (reference out=w140:refnum<vi>, error out=w144:errorcluster, "Value"=w143:dbl)  [unwired: 1 in]
          n93 = property class="DigNum (strict)"(reference=w108) -> (reference out=w110:refnum<vi>, error out=w109:errorcluster, "Value"=w107:dbl)  [unwired: 1 in]
          n94 = property class="DigNum (strict)"(reference=w201) -> (reference out=w200:refnum<vi>, error out=w199:errorcluster, "Value"=w142:dbl)  [unwired: 1 in]
          n95 = property class="DigNum (strict)"(reference=w196) -> (reference out=w197:refnum<vi>, error out=w198:errorcluster, "Value"=w195:dbl)  [unwired: 1 in]
          n96 = property class="DigNum (strict)"(reference=w193) -> (reference out=w191:refnum<vi>, error out=w192:errorcluster, "Value"=w190:dbl)  [unwired: 1 in]
          n97 = property class="DigNum (strict)"(reference=w187) -> (reference out=w189:refnum<vi>, error out=w188:errorcluster, "Value"=w181:dbl)  [unwired: 1 in]
          n98 = property class="DigNum (strict)"(reference=w186) -> (reference out=w184:refnum<vi>, error out=w185:errorcluster, "Value"=w180:dbl)  [unwired: 1 in]
          n99 = property class="DigNum (strict)"(reference=w182) -> (reference out=w179:refnum<vi>, error out=w183:errorcluster, "Value"=w178:dbl)  [unwired: 1 in]
          n100 = property class="DigNum (strict)"(reference=w176) -> (reference out=w177:refnum<vi>, error out=w175:errorcluster, "Value"=w174:dbl)  [unwired: 1 in]
          n101 = property class="DigNum (strict)"(reference=w172) -> (reference out=w171:refnum<vi>, error out=w173:errorcluster, "Value"=w162:dbl)  [unwired: 1 in]
          n102 = property class="DigNum (strict)"(reference=w169) -> (reference out=w170:refnum<vi>, error out=w168:errorcluster, "Value"=w161:dbl)  [unwired: 1 in]
          n103 = property class="DigNum (strict)"(reference=w163) -> (reference out=w160:refnum<vi>, error out=w164:errorcluster, "Value"=w159:dbl)  [unwired: 1 in]
          n104 = Close Reference(reference=w140, error in (no error)=w144) -> ()  [unwired: 1 out]
          n105 = property class="DigNum (strict)"(reference=w113) -> (reference out=w112:refnum<vi>, error out=w114:errorcluster, "Value"=w111:dbl)  [unwired: 1 in]
          n106 = call "ELAPSED TIMER VI FOR REPORT LOOP.vi"("TARGET"=w146, "RESET"=FALSE ("PAUSE"), "PAUSE"=w116) -> ("ELAPSED TIMER"=w203:dbl)  [unwired: 6 in, 2 out]
          n107 = Close Reference(reference=w110, error in (no error)=w109) -> ()  [unwired: 1 out]
          n108 = Build Array(w203) -> (w139:dbl[])
          n109 = Divide(x=w143, y=w142) -> (x/y=w141:dbl)
          n110 = Close Reference(reference=w200, error in (no error)=w199) -> ()  [unwired: 1 out]
          n111 = Close Reference(reference=w197, error in (no error)=w198) -> ()  [unwired: 1 out]
          n112 = Close Reference(reference=w191, error in (no error)=w192) -> ()  [unwired: 1 out]
          n113 = Close Reference(reference=w189, error in (no error)=w188) -> ()  [unwired: 1 out]
          n114 = Close Reference(reference=w184, error in (no error)=w185) -> ()  [unwired: 1 out]
          n115 = Close Reference(reference=w179, error in (no error)=w183) -> ()  [unwired: 1 out]
          n116 = Close Reference(reference=w177, error in (no error)=w175) -> ()  [unwired: 1 out]
          n117 = Close Reference(reference=w171, error in (no error)=w173) -> ()  [unwired: 1 out]
          n118 = Close Reference(reference=w170, error in (no error)=w168) -> ()  [unwired: 1 out]
          n119 = Close Reference(reference=w160, error in (no error)=w164) -> ()  [unwired: 1 out]
          n120 = Close Reference(reference=w112, error in (no error)=w114) -> ()  [unwired: 1 out]
          n121 = Divide(x=w195, y=w142) -> (x/y=w194:dbl)
          n122 = Not(x=w116) -> (.not. x?=w115:bool)
          n123 = Build Array(w142) -> (w138:dbl[])
          n124 = Build Array(w195) -> (w137:dbl[])
          n125 = Build Array(w194) -> (w136:dbl[])
          n126 = Build Array(w190) -> (w135:dbl[])
          n127 = Build Array(w107) -> (w134:dbl[])
          n128 = Build Array(w181) -> (w133:dbl[])
          n129 = Build Array(w180) -> (w132:dbl[])
          n130 = Build Array(w143) -> (w131:dbl[])
          n131 = Build Array(w141) -> (w130:dbl[])
          n132 = Build Array(w178) -> (w129:dbl[])
          n133 = Build Array(w174) -> (w128:dbl[])
          n134 = Build Array(w111) -> (w127:dbl[])
          n135 = Build Array(w162) -> (w126:dbl[])
          n136 = Build Array(w161) -> (w125:dbl[])
          n137 = Build Array(w159) -> (w124:dbl[])
          n138 = Build Array(w158) -> (w123:dbl[])
          n139 = Build Array(w157) -> (w122:dbl[])
          n140 = Build Array(w156) -> (w121:dbl[])
          n141 = Build Array(w85) -> (w120:dbl[])
          n142 = Build Array(w86) -> (w87:dbl[])
          n143 = Build Array(w99) -> (w88:dbl[])
          n144 = Build Array(w106) -> (w89:dbl[])
          n145 = Build Array(w105) -> (w90:dbl[])
          n146 = Build Array(w155) -> (w91:dbl[])
          n147 = Build Array(w154) -> (w92:dbl[])
          n148 = Build Array(w98) -> (w93:dbl[])
          n149 = Build Array(w153) -> (w94:dbl[])
          n150 = Build Array(w152) -> (w95:dbl[])
          n151 = Build Array(w151) -> (w96:dbl[])
          n152 = Build Array(w150) -> (w97:dbl[])
          n153 = Insert Into Array(array=sgl[][] [], new element #1=w139, new element #2=w138, new element #3=w137, new element #4=w136, new element #5=w135, new element #6=w134, new element #7=w133, new element #8=w132, new element #9=w131, new element #10=w130, new element #11=w129, new element #12=w129, new element #13=w128, new element #14=w127, new element #15=w126, new element #16=w125, new element #17=w124, new element #18=w123, new element #19=w122, new element #20=w121, new element #21=w120, new element #22=w87, new element #23=w88, new element #24=w89, new element #25=w90, new element #26=w91, new element #27=w92, new element #28=w93, new element #29=w94, new element #30=w95, new element #31=w96, new element #32=w97) -> (w119:sgl[][])  [unwired: 2 in]
          n154 = case shown="True" w115 {
            tunnel: w119 -> [_ w216]
            frame False {
            }
            frame True {
              n155 = local read "tdms file out"() -> (w215:refnum<k34>)
              n156 = TDMS Write(0:w215, 5:"Measurement" ("group name in (Untitled)"), 7:string[] ["Time(Sec)", "Normal Load (N)", "Friction Force(N)", "Coefficient of Friction", " Depth (Microns)", "Speed (RPM0", "Frequency (Hz)", "Angle (Degree)", "Cyclic Friction Force (N)", "Cyclic Co-Efficient Friction Force", "Stage Temperature (Degree celcius)", "Sample Temperature (Degree celcius)", "Stroke Length (mm)", "Scratch Speed (mm/sec)", "Amb Humidity (%Rh)", "Amb Temperature (Deg C)", "Acoustic (mV)", "Mx(Nm)", "My(Nm)", "Mz (Nm)", "Humidity(%Rh)", "Sliding Distance (mm)", "Wear Track Diameter(mm)", "Fx(N)", "Fy(N)", "MTM Ball Speed(RPM)", "MTM Disc Speed (RPM)", "Entrainment Speed", "Slide Role", "Slip(%)", "Rotart Speed (m/sec)", "MTM Ball Speed (m/sec)", "MTM Disc Speed (m/sec)", "ECR (ohms)"] ("array"), 9:w216) -> (4:w214:refnum<k34>)  [unwired: 2 in, 3 out]
              n157 = local write "tdms file out"(w214) -> ()
            }
          }
          "TDMS CLOSE" <- TRUE ("TDMS CLOSE")
        }
      }
    }
    frame Error {
    }
  }
